vi "shooter_calc.vi"(11 "Shooter":T2) -> (3 "Shooter_Outputs":T1)   [LabVIEW 2012]
uses:
  shooter_cmds.ctl
  shooter_outputs.ctl
panel:
  in  "Shooter LowV":dbl=10.0
  in  "Shooter HighV":dbl=12.0
  in  "Shooter_Outputs 2":T1
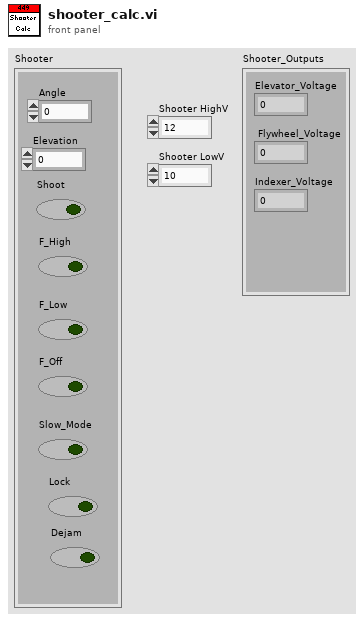
[diagram p1: front panel]
types:
  T1 = typedef "shooter_outputs.ctl" = cluster{"Elevator_Voltage":dbl, " Flywheel_Voltage":dbl, "Indexer_Voltage":dbl}
  T2 = typedef "shooter_cmds.ctl" = cluster{"Elevation":dbl, "Shoot":bool, "F_High":bool, "F_Low":bool, "F_Off":bool, "Slow_Mode":bool, "Lock":bool, "Dejam":bool, "Angle":dbl}
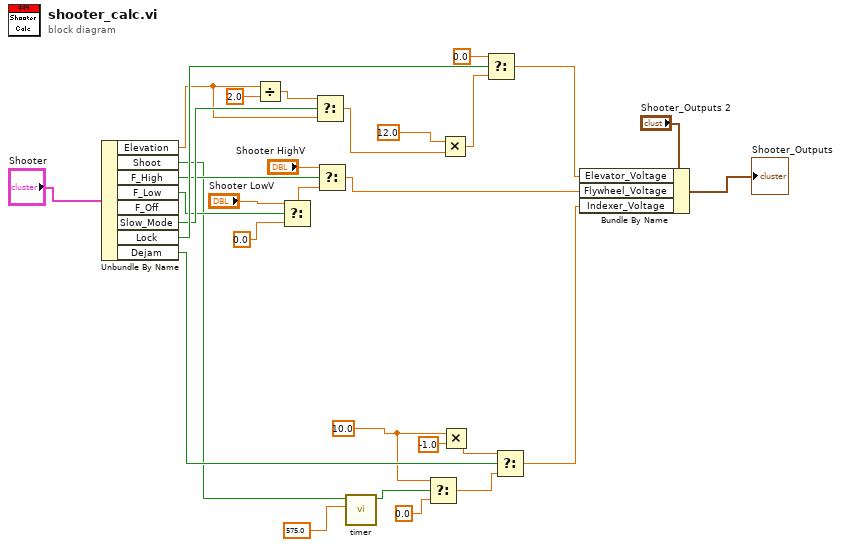
[diagram p0: block diagram]
diagram:
  w2 = 10.0 ("Indexer_Voltage")
  n1 = Unbundle By Name("Shooter") -> ("Elevation"=w19:dbl, "Shoot"=w6:bool, "F_High"=w12:bool, "F_Low"=w13:bool, "Slow_Mode"=w22:bool, "Lock"=w27:bool, "Dejam"=w17:bool)  [unwired: 1 out]
  n2 = Divide(x=w19, y=2.0) -> (x/y=w21:dbl)
  n3 = Select(t="Shooter LowV", s=w13, f=0.0) -> (s? t:f=w11:dbl)
  n4 = Select(t=w21, s=w22, f=w19) -> (s? t:f=w18:dbl)
  n5 = Select(t="Shooter HighV", s=w12, f=w11) -> (s? t:f=w8:dbl)
  n6 = call "timer.vi"("Time"=575.0, "In"=w6) -> ("Out"=w5:bool)  [unwired: 9 in]
  n7 = Select(t=w2, s=w5, f=0.0) -> (s? t:f=w4:dbl)
  n8 = Multiply(x=12.0, y=w18) -> (x*y=w25:dbl)
  n9 = Multiply(x=w2, y=-1.0) -> (x*y=w16:dbl)
  n10 = Select(t=0.0, s=w27, f=w25) -> (s? t:f=w26:dbl)
  n11 = Select(t=w16, s=w17, f=w4) -> (s? t:f=w14:dbl)
  n12 = Bundle By Name(cluster="Shooter_Outputs 2", "Elevator_Voltage"=w26, "Flywheel_Voltage"=w8, "Indexer_Voltage"=w14) -> (→"Shooter_Outputs":T1)
